vi "FGV Amium Daten.vi"(0 "Amium Komm  Daten":T8, 1 "Grenzwerte PNS":T1={"Filter:"={"Sollwert"=0.0, "Warn-Min"=0.0, "Warn-Max"=0.0, "Abschalt-Min"=0.0, "Abschalt-Max"=0.0, "Regler"=1}, "Ventilplatte:"={"Sollwert"=0.0, "Warn-Min"=0.0, "Warn-Max"=0.0, "Abschalt-Min"=0.0, "Abschalt-Max"=0.0, "Regler"=1}, "Heizleitung 1:"={"Sollwert"=0.0, "Warn-Min"=0.0, "Warn-Max"=0.0, "Abschalt-Min"=0.0, "Abschalt-Max"=0.0, "Regler"=1}, "Heizleitung 2:"={"Sollwert"=0.0, "Warn-Min"=0.0, "Warn-Max"=0.0, "Abschalt-Min"=0.0, "Abschalt-Max"=0.0, "Regler"=1}, "Heizleitung 3:"={"Sollwert"=0.0, "Warn-Min"=0.0, "Warn-Max"=0.0, "Abschalt-Min"=0.0, "Abschalt-Max"=0.0, "Regler"=1}, "Heizleitung 4:"={"Sollwert"=0.0, "Warn-Min"=0.0, "Warn-Max"=0.0, "Abschalt-Min"=0.0, "Abschalt-Max"=0.0, "Regler"=1}, "Heizleitung 5:"={"Sollwert"=0.0, "Warn-Min"=0.0, "Warn-Max"=0.0, "Abschalt-Min"=0.0, "Abschalt-Max"=0.0, "Regler"=1}, "Heizleitung 6:"={"Sollwert"=0.0, "Warn-Min"=0.0, "Warn-Max"=0.0, "Abschalt-Min"=0.0, "Abschalt-Max"=0.0, "Regler"=1}, "Heizleitung 7:"={"Sollwert"=0.0, "Warn-Min"=0.0, "Warn-Max"=0.0, "Abschalt-Min"=0.0, "Abschalt-Max"=1.0, "Regler"=1}, "Heizleitung 8:"={"Sollwert"=0.0, "Warn-Min"=0.0, "Warn-Max"=0.0, "Abschalt-Min"=0.0, "Abschalt-Max"=0.0, "Regler"=1}, "Heizleitung 9:"={"Sollwert"=0.0, "Warn-Min"=0.0, "Warn-Max"=0.0, "Abschalt-Min"=0.0, "Abschalt-Max"=0.0, "Regler"=1}, "Heizleitung 10:"={"Sollwert"=0.0, "Warn-Min"=0.0, "Warn-Max"=0.0, "Abschalt-Min"=0.0, "Abschalt-Max"=0.0, "Regler"=1}, "Heizleitung 11:"={"Sollwert"=0.0, "Warn-Min"=0.0, "Warn-Max"=0.0, "Abschalt-Min"=0.0, "Abschalt-Max"=0.0, "Regler"=1}, "Heizleitung 12:"={"Sollwert"=0.0, "Warn-Min"=0.0, "Warn-Max"=0.0, "Abschalt-Min"=0.0, "Abschalt-Max"=0.0, "Regler"=1}} {"Heizleitung 12:"."Regler" items=["aktiv", "inaktiv"]; "Heizleitung 12:"."Abschalt-Max" format="%#_5g"; "Heizleitung 12:"."Abschalt-Min" format="%#_5g"; "Heizleitung 12:"."Warn-Max" format="%#_5g"; "Heizleitung 12:"."Warn-Min" format="%#_5g"; "Heizleitung 12:"."Sollwert" format="%#_5g"; "Heizleitung 11:"."Regler" items=["aktiv", "inaktiv"]; "Heizleitung 11:"."Abschalt-Max" format="%#_5g"; "Heizleitung 11:"."Abschalt-Min" format="%#_5g"; "Heizleitung 11:"."Warn-Max" format="%#_5g"; "Heizleitung 11:"."Warn-Min" format="%#_5g"; "Heizleitung 11:"."Sollwert" format="%#_5g"; "Heizleitung 10:"."Regler" items=["aktiv", "inaktiv"]; "Heizleitung 10:"."Abschalt-Max" format="%#_5g"; "Heizleitung 10:"."Abschalt-Min" format="%#_5g"; "Heizleitung 10:"."Warn-Max" format="%#_5g"; "Heizleitung 10:"."Warn-Min" format="%#_5g"; "Heizleitung 10:"."Sollwert" format="%#_5g"; "Heizleitung 9:"."Regler" items=["aktiv", "inaktiv"]; "Heizleitung 9:"."Abschalt-Max" format="%#_5g"; "Heizleitung 9:"."Abschalt-Min" format="%#_5g"; "Heizleitung 9:"."Warn-Max" format="%#_5g"; "Heizleitung 9:"."Warn-Min" format="%#_5g"; "Heizleitung 9:"."Sollwert" format="%#_5g"; "Heizleitung 8:"."Regler" items=["aktiv", "inaktiv"]; "Heizleitung 8:"."Abschalt-Max" format="%#_5g"; "Heizleitung 8:"."Abschalt-Min" format="%#_5g"; "Heizleitung 8:"."Warn-Max" format="%#_5g"; "Heizleitung 8:"."Warn-Min" format="%#_5g"; "Heizleitung 8:"."Sollwert" format="%#_5g"; "Heizleitung 7:"."Regler" items=["aktiv", "inaktiv"]; "Heizleitung 7:"."Abschalt-Max" format="%#_5g"; "Heizleitung 7:"."Abschalt-Min" format="%#_5g"; "Heizleitung 7:"."Warn-Max" format="%#_5g"; "Heizleitung 7:"."Warn-Min" format="%#_5g"; "Heizleitung 7:"."Sollwert" format="%#_5g"; "Heizleitung 6:"."Regler" items=["aktiv", "inaktiv"]; "Heizleitung 6:"."Abschalt-Max" format="%#_5g"; "Heizleitung 6:"."Abschalt-Min" format="%#_5g"; "Heizleitung 6:"."Warn-Max" format="%#_5g"; "Heizleitung 6:"."Warn-Min" format="%#_5g"; "Heizleitung 6:"."Sollwert" format="%#_5g"; "Heizleitung 5:"."Regler" items=["aktiv", "inaktiv"]; "Heizleitung 5:"."Abschalt-Max" format="%#_5g"; "Heizleitung 5:"."Abschalt-Min" format="%#_5g"; "Heizleitung 5:"."Warn-Max" format="%#_5g"; "Heizleitung 5:"."Warn-Min" format="%#_5g"; "Heizleitung 5:"."Sollwert" format="%#_5g"; "Heizleitung 4:"."Regler" items=["aktiv", "inaktiv"]; "Heizleitung 4:"."Abschalt-Max" format="%#_5g"; "Heizleitung 4:"."Abschalt-Min" format="%#_5g"; "Heizleitung 4:"."Warn-Max" format="%#_5g"; "Heizleitung 4:"."Warn-Min" format="%#_5g"; "Heizleitung 4:"."Sollwert" format="%#_5g"; "Heizleitung 3:"."Regler" items=["aktiv", "inaktiv"]; "Heizleitung 3:"."Abschalt-Max" format="%#_5g"; "Heizleitung 3:"."Abschalt-Min" format="%#_5g"; "Heizleitung 3:"."Warn-Max" format="%#_5g"; "Heizleitung 3:"."Warn-Min" format="%#_5g"; "Heizleitung 3:"."Sollwert" format="%#_5g"; "Heizleitung 2:"."Regler" items=["aktiv", "inaktiv"]; "Heizleitung 2:"."Abschalt-Max" format="%#_5g"; "Heizleitung 2:"."Abschalt-Min" format="%#_5g"; "Heizleitung 2:"."Warn-Max" format="%#_5g"; "Heizleitung 2:"."Warn-Min" format="%#_5g"; "Heizleitung 2:"."Sollwert" format="%#_5g"; "Heizleitung 1:"."Regler" items=["aktiv", "inaktiv"]; "Heizleitung 1:"."Abschalt-Max" format="%#_5g"; "Heizleitung 1:"."Abschalt-Min" format="%#_5g"; "Heizleitung 1:"."Warn-Max" format="%#_5g"; "Heizleitung 1:"."Warn-Min" format="%#_5g"; "Heizleitung 1:"."Sollwert" format="%#_5g"; "Ventilplatte:"."Regler" items=["aktiv", "inaktiv"]; "Ventilplatte:"."Abschalt-Max" format="%#_5g"; "Ventilplatte:"."Abschalt-Min" format="%#_5g"; "Ventilplatte:"."Warn-Max" format="%#_5g"; "Ventilplatte:"."Warn-Min" format="%#_5g"; "Ventilplatte:"."Sollwert" format="%#_5g"; "Filter:"."Regler" items=["aktiv", "inaktiv"]; "Filter:"."Abschalt-Max" format="%#_5g"; "Filter:"."Abschalt-Min" format="%#_5g"; "Filter:"."Warn-Max" format="%#_5g"; "Filter:"."Warn-Min" format="%#_5g"; "Filter:"."Sollwert" format="%#_5g"}, 5 "Amium Daten":T6 {"Amium Zustände" items=["Pause", "Aufheizphase", "Standby", "Messen", "Spülen", "Leakcheck"]}, 7 "Fehler Cluster":T5, 9 "Regler":T4[](array[typedef]) {"Error" format="%#.0f"; "Status" format="%#.0f"; "Stellgröße" format="%#.0f"; "Sollwert" format="%#.0f"; "Istwert" format="%#.0f"}, 11 "error in (no error)":errorcluster caption="Fehler (Eingang, kein Fehler)", 13 "Aktion":T9) -> (3 "Grenzwerte PNS":T1={"Filter:"={"Sollwert"=0.0, "Warn-Min"=0.0, "Warn-Max"=0.0, "Abschalt-Min"=0.0, "Abschalt-Max"=0.0, "Regler"=1}, "Ventilplatte:"={"Sollwert"=0.0, "Warn-Min"=0.0, "Warn-Max"=0.0, "Abschalt-Min"=0.0, "Abschalt-Max"=0.0, "Regler"=1}, "Heizleitung 1:"={"Sollwert"=0.0, "Warn-Min"=0.0, "Warn-Max"=0.0, "Abschalt-Min"=0.0, "Abschalt-Max"=0.0, "Regler"=1}, "Heizleitung 2:"={"Sollwert"=0.0, "Warn-Min"=0.0, "Warn-Max"=0.0, "Abschalt-Min"=0.0, "Abschalt-Max"=0.0, "Regler"=1}, "Heizleitung 3:"={"Sollwert"=0.0, "Warn-Min"=0.0, "Warn-Max"=0.0, "Abschalt-Min"=0.0, "Abschalt-Max"=0.0, "Regler"=1}, "Heizleitung 4:"={"Sollwert"=0.0, "Warn-Min"=0.0, "Warn-Max"=0.0, "Abschalt-Min"=0.0, "Abschalt-Max"=0.0, "Regler"=1}, "Heizleitung 5:"={"Sollwert"=0.0, "Warn-Min"=0.0, "Warn-Max"=0.0, "Abschalt-Min"=0.0, "Abschalt-Max"=0.0, "Regler"=1}, "Heizleitung 6:"={"Sollwert"=0.0, "Warn-Min"=0.0, "Warn-Max"=0.0, "Abschalt-Min"=0.0, "Abschalt-Max"=0.0, "Regler"=1}, "Heizleitung 7:"={"Sollwert"=0.0, "Warn-Min"=0.0, "Warn-Max"=0.0, "Abschalt-Min"=0.0, "Abschalt-Max"=1.0, "Regler"=1}, "Heizleitung 8:"={"Sollwert"=0.0, "Warn-Min"=0.0, "Warn-Max"=0.0, "Abschalt-Min"=0.0, "Abschalt-Max"=0.0, "Regler"=1}, "Heizleitung 9:"={"Sollwert"=0.0, "Warn-Min"=0.0, "Warn-Max"=0.0, "Abschalt-Min"=0.0, "Abschalt-Max"=0.0, "Regler"=1}, "Heizleitung 10:"={"Sollwert"=0.0, "Warn-Min"=0.0, "Warn-Max"=0.0, "Abschalt-Min"=0.0, "Abschalt-Max"=0.0, "Regler"=1}, "Heizleitung 11:"={"Sollwert"=0.0, "Warn-Min"=0.0, "Warn-Max"=0.0, "Abschalt-Min"=0.0, "Abschalt-Max"=0.0, "Regler"=1}, "Heizleitung 12:"={"Sollwert"=0.0, "Warn-Min"=0.0, "Warn-Max"=0.0, "Abschalt-Min"=0.0, "Abschalt-Max"=0.0, "Regler"=1}} {"Heizleitung 12:"."Regler" items=["aktiv", "inaktiv"]; "Heizleitung 12:"."Abschalt-Max" format="%#_5g"; "Heizleitung 12:"."Abschalt-Min" format="%#_5g"; "Heizleitung 12:"."Warn-Max" format="%#_5g"; "Heizleitung 12:"."Warn-Min" format="%#_5g"; "Heizleitung 12:"."Sollwert" format="%#_5g"; "Heizleitung 11:"."Regler" items=["aktiv", "inaktiv"]; "Heizleitung 11:"."Abschalt-Max" format="%#_5g"; "Heizleitung 11:"."Abschalt-Min" format="%#_5g"; "Heizleitung 11:"."Warn-Max" format="%#_5g"; "Heizleitung 11:"."Warn-Min" format="%#_5g"; "Heizleitung 11:"."Sollwert" format="%#_5g"; "Heizleitung 10:"."Regler" items=["aktiv", "inaktiv"]; "Heizleitung 10:"."Abschalt-Max" format="%#_5g"; "Heizleitung 10:"."Abschalt-Min" format="%#_5g"; "Heizleitung 10:"."Warn-Max" format="%#_5g"; "Heizleitung 10:"."Warn-Min" format="%#_5g"; "Heizleitung 10:"."Sollwert" format="%#_5g"; "Heizleitung 9:"."Regler" items=["aktiv", "inaktiv"]; "Heizleitung 9:"."Abschalt-Max" format="%#_5g"; "Heizleitung 9:"."Abschalt-Min" format="%#_5g"; "Heizleitung 9:"."Warn-Max" format="%#_5g"; "Heizleitung 9:"."Warn-Min" format="%#_5g"; "Heizleitung 9:"."Sollwert" format="%#_5g"; "Heizleitung 8:"."Regler" items=["aktiv", "inaktiv"]; "Heizleitung 8:"."Abschalt-Max" format="%#_5g"; "Heizleitung 8:"."Abschalt-Min" format="%#_5g"; "Heizleitung 8:"."Warn-Max" format="%#_5g"; "Heizleitung 8:"."Warn-Min" format="%#_5g"; "Heizleitung 8:"."Sollwert" format="%#_5g"; "Heizleitung 7:"."Regler" items=["aktiv", "inaktiv"]; "Heizleitung 7:"."Abschalt-Max" format="%#_5g"; "Heizleitung 7:"."Abschalt-Min" format="%#_5g"; "Heizleitung 7:"."Warn-Max" format="%#_5g"; "Heizleitung 7:"."Warn-Min" format="%#_5g"; "Heizleitung 7:"."Sollwert" format="%#_5g"; "Heizleitung 6:"."Regler" items=["aktiv", "inaktiv"]; "Heizleitung 6:"."Abschalt-Max" format="%#_5g"; "Heizleitung 6:"."Abschalt-Min" format="%#_5g"; "Heizleitung 6:"."Warn-Max" format="%#_5g"; "Heizleitung 6:"."Warn-Min" format="%#_5g"; "Heizleitung 6:"."Sollwert" format="%#_5g"; "Heizleitung 5:"."Regler" items=["aktiv", "inaktiv"]; "Heizleitung 5:"."Abschalt-Max" format="%#_5g"; "Heizleitung 5:"."Abschalt-Min" format="%#_5g"; "Heizleitung 5:"."Warn-Max" format="%#_5g"; "Heizleitung 5:"."Warn-Min" format="%#_5g"; "Heizleitung 5:"."Sollwert" format="%#_5g"; "Heizleitung 4:"."Regler" items=["aktiv", "inaktiv"]; "Heizleitung 4:"."Abschalt-Max" format="%#_5g"; "Heizleitung 4:"."Abschalt-Min" format="%#_5g"; "Heizleitung 4:"."Warn-Max" format="%#_5g"; "Heizleitung 4:"."Warn-Min" format="%#_5g"; "Heizleitung 4:"."Sollwert" format="%#_5g"; "Heizleitung 3:"."Regler" items=["aktiv", "inaktiv"]; "Heizleitung 3:"."Abschalt-Max" format="%#_5g"; "Heizleitung 3:"."Abschalt-Min" format="%#_5g"; "Heizleitung 3:"."Warn-Max" format="%#_5g"; "Heizleitung 3:"."Warn-Min" format="%#_5g"; "Heizleitung 3:"."Sollwert" format="%#_5g"; "Heizleitung 2:"."Regler" items=["aktiv", "inaktiv"]; "Heizleitung 2:"."Abschalt-Max" format="%#_5g"; "Heizleitung 2:"."Abschalt-Min" format="%#_5g"; "Heizleitung 2:"."Warn-Max" format="%#_5g"; "Heizleitung 2:"."Warn-Min" format="%#_5g"; "Heizleitung 2:"."Sollwert" format="%#_5g"; "Heizleitung 1:"."Regler" items=["aktiv", "inaktiv"]; "Heizleitung 1:"."Abschalt-Max" format="%#_5g"; "Heizleitung 1:"."Abschalt-Min" format="%#_5g"; "Heizleitung 1:"."Warn-Max" format="%#_5g"; "Heizleitung 1:"."Warn-Min" format="%#_5g"; "Heizleitung 1:"."Sollwert" format="%#_5g"; "Ventilplatte:"."Regler" items=["aktiv", "inaktiv"]; "Ventilplatte:"."Abschalt-Max" format="%#_5g"; "Ventilplatte:"."Abschalt-Min" format="%#_5g"; "Ventilplatte:"."Warn-Max" format="%#_5g"; "Ventilplatte:"."Warn-Min" format="%#_5g"; "Ventilplatte:"."Sollwert" format="%#_5g"; "Filter:"."Regler" items=["aktiv", "inaktiv"]; "Filter:"."Abschalt-Max" format="%#_5g"; "Filter:"."Abschalt-Min" format="%#_5g"; "Filter:"."Warn-Max" format="%#_5g"; "Filter:"."Warn-Min" format="%#_5g"; "Filter:"."Sollwert" format="%#_5g"}, 4 "Amium Komm Daten":T8, 6 "Amium Daten":T6 {"Amium Zustände" items=["Pause", "Aufheizphase", "Standby", "Messen", "Spülen", "Leakcheck"]}, 8 "Fehler Cluster":T5, 10 "Regler":T4[](array[typedef]) {"Error" format="%#.0f"; "Status" format="%#.0f"; "Stellgröße" format="%#.0f"; "Sollwert" format="%#.0f"; "Istwert" format="%#.0f"}, 15 "error out":errorcluster caption="Fehler (Ausgang)")   [LabVIEW 2020, in "Amium PNS.lvlib"]
uses:
  Amium PNS.lvlib
  Aktion FGV Amium Daten.ctl
  Kommunikation Daten Cluster.ctl
  Daten Cluster.ctl
  Amium Zustand.ctl
  Amium ErrorCluster.ctl
  Temperaturregler Cluster.ctl
  Amium Anlagengrenzwerte PNS.ctl
  Amium Anlagengrenzwerte-Parameter Anzeige.ctl
  Visualisierungs Elemente/Zahlen-Eingabefeld.ctl
  Allgemein/allgemeine Sub-VIs.lvlib
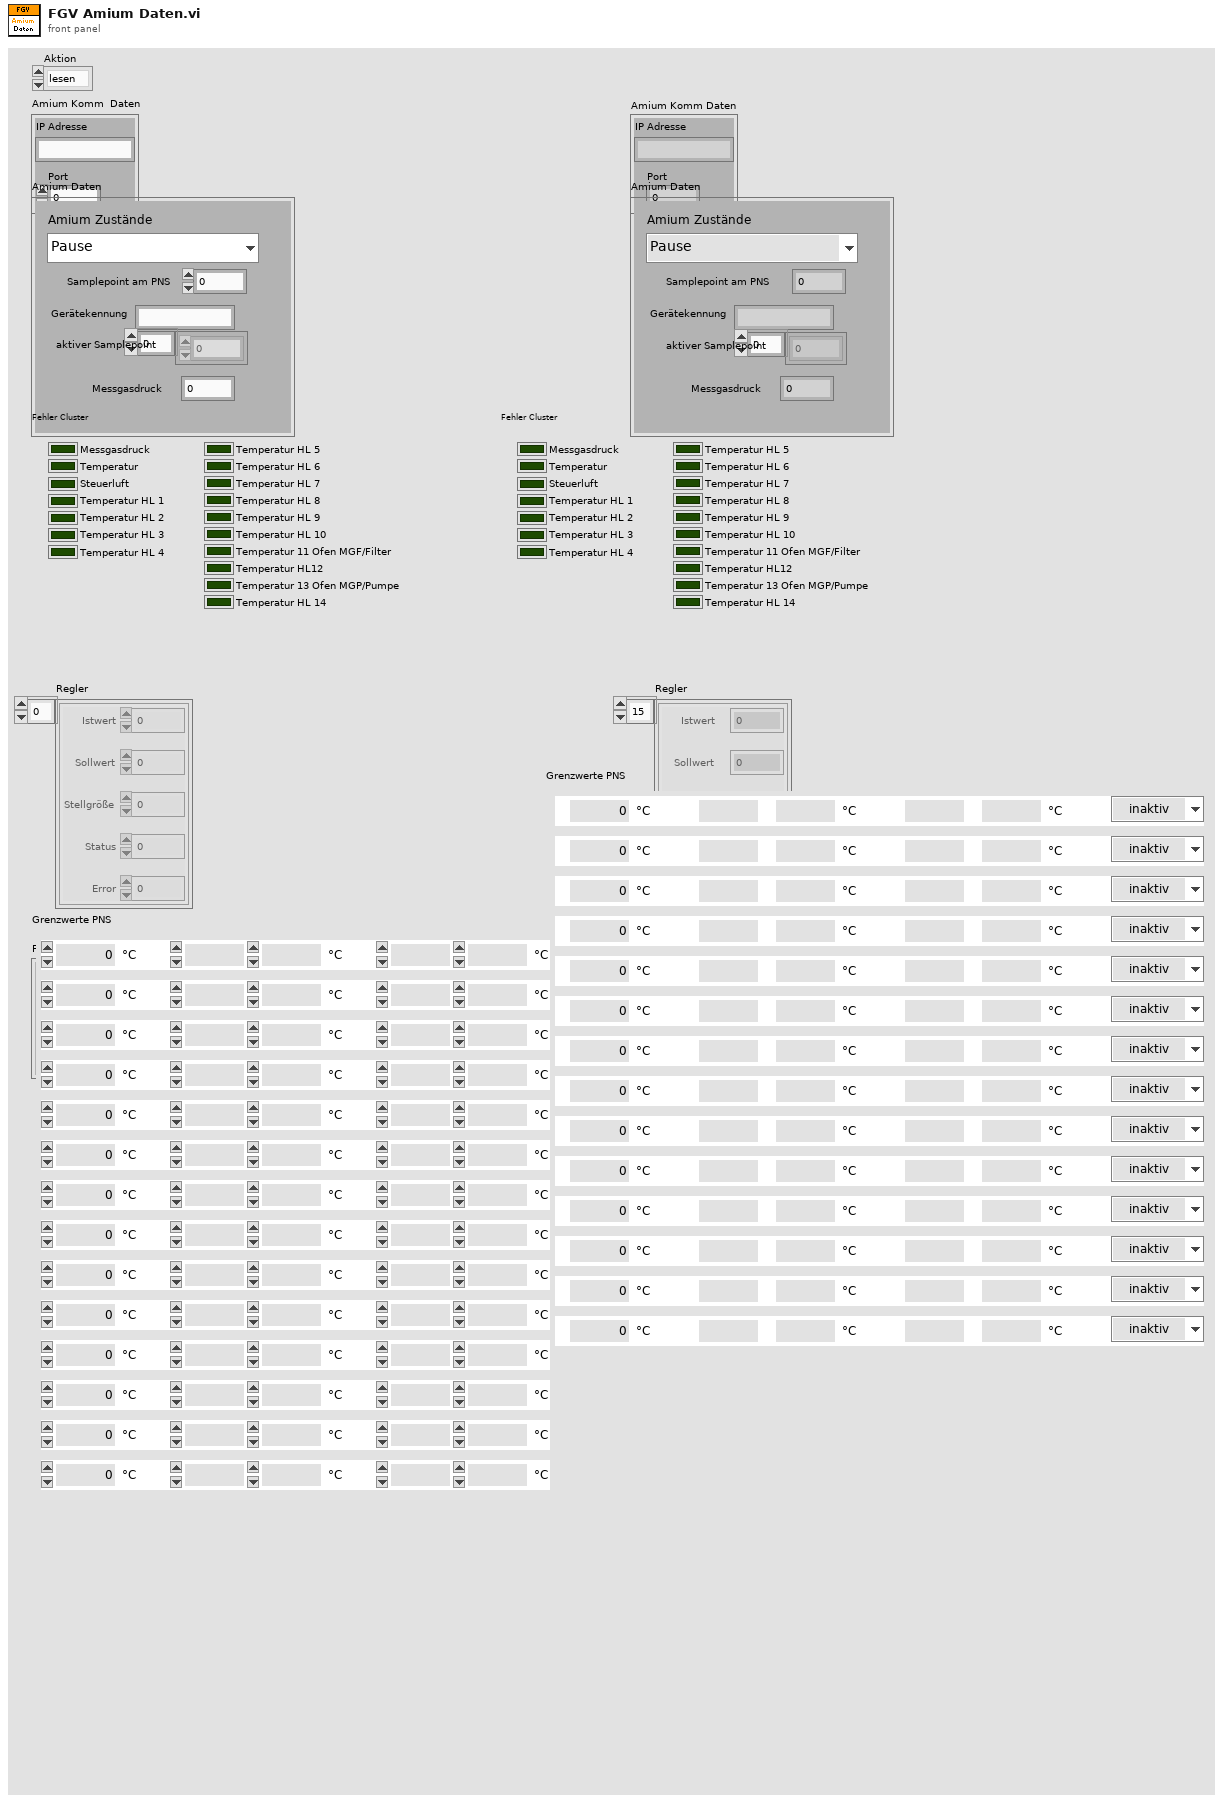
[diagram p1: front panel]
types:
  T1 = typedef "Amium PNS.lvlib/Amium Anlagengrenzwerte PNS.ctl" = cluster{"Filter:":T2, "Ventilplatte:":T2, "Heizleitung 1:":T2, "Heizleitung 2:":T2, "Heizleitung 3:":T2, "Heizleitung 4:":T2, "Heizleitung 5:":T2, "Heizleitung 6:":T2, "Heizleitung 7:":T2, "Heizleitung 8:":T2, "Heizleitung 9:":T2, "Heizleitung 10:":T2, "Heizleitung 11:":T2, "Heizleitung 12:":T2}
  T2 = typedef "Amium PNS.lvlib/Amium Anlagengrenzwerte-Parameter Anzeige.ctl" = cluster{"Sollwert":T3, "Warn-Min":T3, "Warn-Max":T3, "Abschalt-Min":T3, "Abschalt-Max":T3, "Regler":u16}
  T3 = typedef "Zahlen-Eingabefeld.ctl" = sgl
  T4 = typedef "Amium PNS.lvlib/Temperaturregler Cluster.ctl" = cluster{"Istwert":sgl, "Sollwert":sgl, "Stellgröße":sgl, "Status":sgl, "Error":sgl}
  T5 = typedef "Amium PNS.lvlib/Amium ErrorCluster.ctl" = cluster{"Messgasdruck":bool, "Temperatur":bool, "Steuerluft":bool, "Temperatur HL 1":bool, "Temperatur HL 2":bool, "Temperatur HL 3":bool, "Temperatur HL 4":bool, "Temperatur HL 5":bool, "Temperatur HL 6":bool, "Temperatur HL 7":bool, "Temperatur HL 8":bool, "Temperatur HL 9":bool, "Temperatur HL 10":bool, "Temperatur 11 Ofen MGF/Filter":bool, "Temperatur HL12":bool, "Temperatur 13 Ofen MGP/Pumpe":bool, "Temperatur HL 14":bool}
  T6 = typedef "Amium PNS.lvlib/Daten Cluster.ctl" = cluster{"Amium Zustände":T7, "Samplepoint am PNS":i16, "Gerätekennung":string, "aktiver Samplepoint":i16[], "Messgasdruck":sgl}
  T7 = typedef "Amium PNS.lvlib/Amium Zustand.ctl" = u16
  T8 = typedef "Amium PNS.lvlib/Kommunikation Daten Cluster.ctl" = cluster{"IP Adresse":string, "Port":i16}
  T9 = typedef "Amium PNS.lvlib/Aktion FGV Amium Daten.ctl" = enum16{"lesen", "Komm Daten", "Daten", "Error", "Regler", "Grenzwerte", "laden", "speichern"}
  T10 = cluster{"[0]":T2, "[1]":T2, "[2]":T2, "[3]":T2, "[4]":T2, "[5]":T2, "[6]":T2, "[7]":T2, "[8]":T2, "[9]":T2, "[10]":T2, "[11]":T2, "[12]":T2, "[13]":T2}
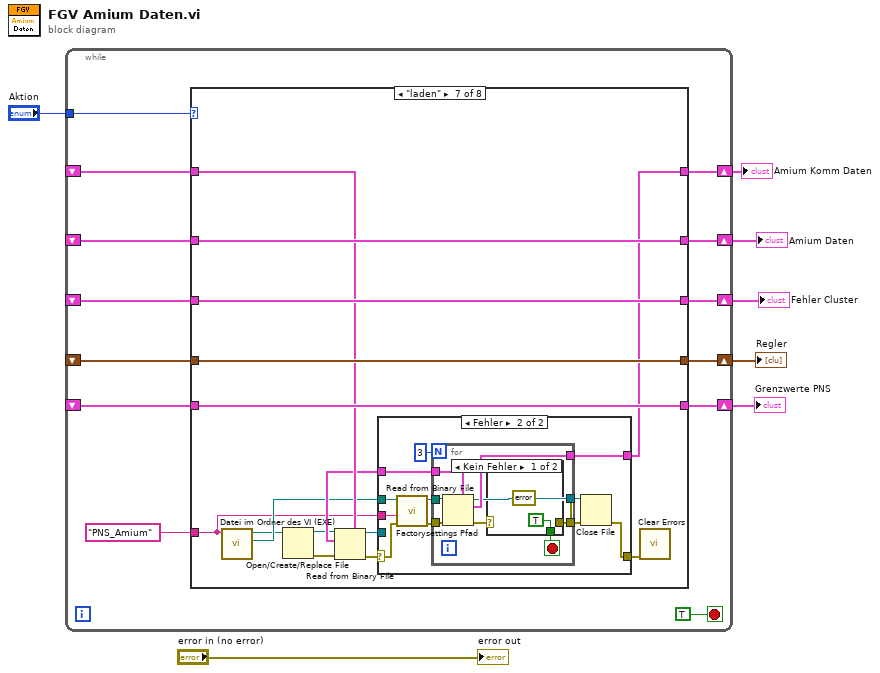
[diagram p0: block diagram]
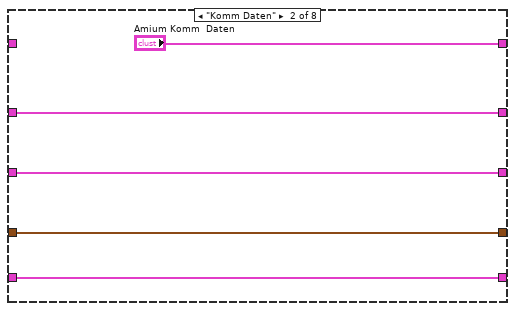
[diagram p3: hidden frame]
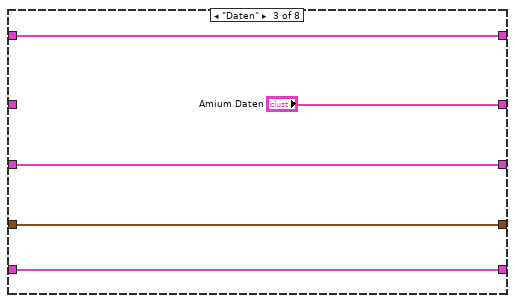
[diagram p4: hidden frame]
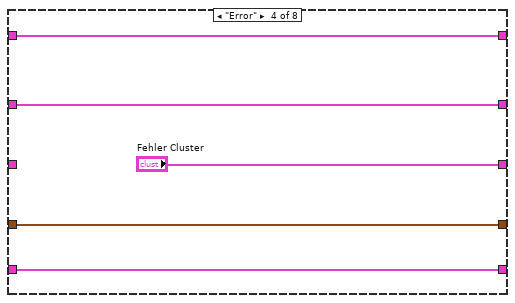
[diagram p5: hidden frame]
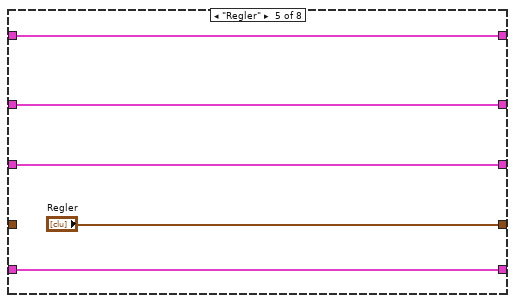
[diagram p6: hidden frame]
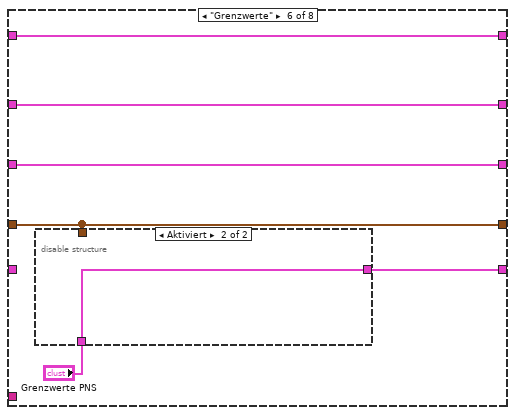
[diagram p7: hidden frame]
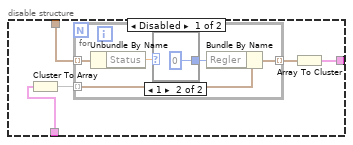
[diagram p8: hidden frame]
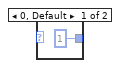
[diagram p9: hidden frame]
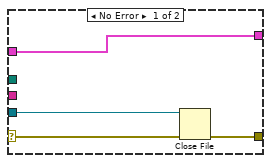
[diagram p10: hidden frame]
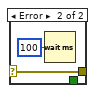
[diagram p11: hidden frame]
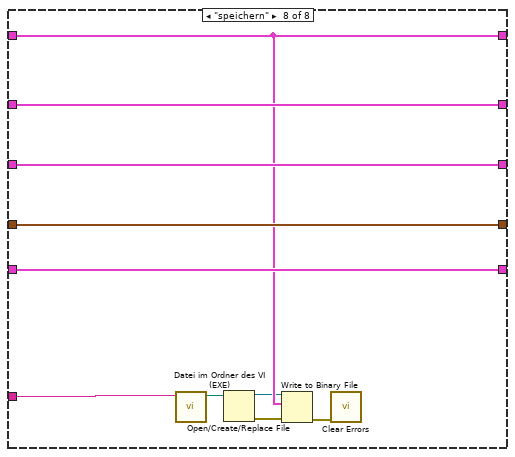
[diagram p12: hidden frame]
diagram:
  n1 = while {
    tunnel: "Aktion" -> [w19]
    shift-right: [w18] -> w6
    shift-left: _ -> [w17]
    shift-right: [w16] -> w4
    shift-left: _ -> [w15]
    shift-right: [w14] -> w3
    shift-left: _ -> [w13]
    shift-right: [w12] -> w2
    shift-left: _ -> [w11]
    shift-right: [w10] -> w1
    shift-left: _ -> [w9]
    stop <- TRUE stop-if-true
    n2 = case shown="\"laden\"" w19 {
      tunnel: [w25 "Amium Komm  Daten" w35 w40 w45 w51 w68 w110] -> w18
      tunnel: w17 -> [w25 _ w35 w40 w45 w51 w75 w110]
      tunnel: [w24 w29 "Amium Daten" w39 w44 w50 w79 w116] -> w16
      tunnel: w15 -> [w24 w29 _ w39 w44 w50 w79 w116]
      tunnel: [w23 w28 w33 "Fehler Cluster" w43 w49 w78 w115] -> w14
      tunnel: w13 -> [w23 w28 w33 _ w43 w49 w78 w115]
      tunnel: [w22 w27 w32 w37 "Regler" w48 w77 w114] -> w12
      tunnel: w11 -> [w22 w27 w32 w37 _ w48 w77 w114]
      tunnel: [w21 w26 w31 w36 w41 w47 w76 w113] -> w10
      tunnel: w9 -> [w21 w26 w31 w36 w41 _ w76 w113]
      tunnel: "PNS_Amium" ("Dateiname") -> [_ _ _ _ _ _ w70 w111]
      frame "lesen", Default {
      }
      frame "Komm Daten" {
      }
      frame "Daten" {
      }
      frame "Error" {
      }
      frame "Regler" {
      }
      frame "Grenzwerte" {
        n3 = disable-structure shown="Aktiviert" {
          disable-tunnel: w48 -> [w56 _]
          disable-tunnel: [w54 w64] -> w47
          disable-tunnel: "Grenzwerte PNS" -> [w52 w64]
          frame Disabled {
            n4 = Cluster To Array(cluster=w52) -> (array=w53:T2[])
            n5 = for {
              tunnel: w56 -> [w61] mode=indexing
              tunnel: w53 -> [w60] mode=indexing
              tunnel: [w59] -> w55 mode=indexing
              n6 = Unbundle By Name(w61) -> ("Status"=w58:sgl)
              n7 = case shown="1" w58 {
                tunnel: [u16 1 ("Regler") u16 0 ("Regler")] -> w57
                frame 0, Default {
                }
                frame 1 {
                }
              }
              n8 = Bundle By Name(cluster=w60, "Regler"=w57) -> (w59:T2)
            }
            n9 = Array To Cluster(array=w55) -> (cluster=w54:T10)
          }
          frame Enabled {
          }
        }
      }
      frame "laden" {
        n10 = call "Datei im Ordner des VI (EXE).vi"("Dateiname"=w70) -> ("Ordner des Haupt-VIs"=w71:path, "Dateipfad im Ordner des Haupt-VIs"=w66:path)  [unwired: 8 in, 1 out]
        n11 = Open/Create/Replace File(file path (use dialog)=w66) -> (refnum out=w65:refnum<file>, error out=w67:errorcluster)  [unwired: 5 in, 1 out]
        n12 = Read from Binary File(5:w75, 8:w67, 11:w65) -> (0:w74:errorcluster, 2:w72:T8, 3:w69:refnum<file>)  [unwired: 4 out]
        n13 = case shown="Fehler" w74 {
          selector: w74 -> [w82 w86]
          tunnel: w71 -> [_ w87]
          tunnel: w72 -> [w83 w85]
          tunnel: [w83 w93] -> w68
          tunnel: [w80 w91] -> w73
          tunnel: w69 -> [w81 _]
          tunnel: w70 -> [_ w84]
          frame No Error {
            n14 = Close File(refnum=w81, error in=w82) -> (error out=w80:errorcluster)  [unwired: 1 out]
          }
          frame Error {
            n15 = call "Factorysettings Pfad.vi"("error in (no error)"=w86, "Dateiname"=w84, "Ordner des Haupt-VIs"=w87) -> ("error out"=w88:errorcluster, "Pfad Factorysettings"=w89:path)  [unwired: 7 in]
            n16 = for {
              N: 3 -> [_]
              tunnel: w88 -> [w100]
              tunnel: w89 -> [w99]
              tunnel: [w98] -> w93
              tunnel: [w97] -> w92
              tunnel: [w96] -> w90
              tunnel: w85 -> [w95]
              stop <- w101 stop-if-true
              n17 = Read from Binary File(5:w95, 8:w100, 11:w99) -> (0:w102:errorcluster, 2:w98:T8, 3:w96:refnum<file>)  [unwired: 3 in, 1 out]
              n18 = case shown="Kein Fehler" w102 {
                selector: w102 -> [_ w105]
                tunnel: [TRUE _] -> w101
                tunnel: [errorcluster {"status"=FALSE, "code"=0, "source"=""} ("error IO") w105] -> w97
                frame No Error {
                }
                frame Error {
                  n19 = Wait (ms)(milliseconds to wait=u32 100 ("Zu wartende ms")) -> ()  [unwired: 1 out]
                }
              }
            }
            n20 = Close File(refnum=w90, error in=w92) -> (error out=w91:errorcluster)  [unwired: 1 out]
          }
        }
        n21 = call <vilib>:"Clear Errors.vi"("error in (no error)"=w73) -> ()  [unwired: 5 in, 2 out]
      }
      frame "speichern" {
        n22 = call "Datei im Ordner des VI (EXE).vi"("Dateiname"=w111) -> ("Dateipfad im Ordner des Haupt-VIs"=w109:path)  [unwired: 8 in, 2 out]
        n23 = Open/Create/Replace File(file path (use dialog)=w109) -> (refnum out=w108:refnum<file>, error out=w107:errorcluster)  [unwired: 5 in, 1 out]
        n24 = Write to Binary File(file (use dialog)=w108, data=w110, error in=w107) -> (error out=w112:errorcluster)  [unwired: 5 out]
        n25 = call <vilib>:"Clear Errors.vi"("error in (no error)"=w112) -> ()  [unwired: 5 in, 2 out]
      }
    }
  }
  "Amium Komm Daten" <- w6
  "Amium Daten" <- w4
  "Fehler Cluster" <- w3
  "Regler" <- w2
  "Grenzwerte PNS" <- w1
  "error out" <- "error in (no error)"
